vi "sub_e-top.vi"(10 "TIM_XYZ_DATA":cluster{"x":sgl, "y":sgl, "Z":sgl}[](array[cluster])=[{"x"=-0.27294323, "y"=0.40705678, "Z"=2.3861455e-08}, {"x"=-0.26954788, "y"=0.41357002, "Z"=2.3564624e-08}, {"x"=-0.26465562, "y"=0.42143202, "Z"=2.3136929e-08}, {"x"=-0.26040056, "y"=0.42853323, "Z"=2.276494e-08}, {"x"=-0.25317857, "y"=0.43833783, "Z"=2.2133573e-08}, {"x"=-0.24585162, "y"=0.4480496, "Z"=2.1493031e-08}, {"x"=-0.26621187, "y"=0.43175167, "Z"=2.327298e-08}, {"x"=-0.27206331, "y"=0.42923805, "Z"=2.378453e-08}, {"x"=-0.27573514, "y"=0.4288046, "Z"=2.4105532e-08}, {"x"=-0.278678, "y"=0.4290746, "Z"=2.4362805e-08}, {"x"=-0.27714488, "y"=0.43335915, "Z"=2.4228775e-08}, {"x"=-0.27406967, "y"=0.43893814, "Z"=2.3959931e-08}, {"x"=-0.2113174, "y"=0.496302, "Z"=1.8473955e-08}, {"x"=-0.14184111, "y"=0.558139, "Z"=1.2400144e-08}, {"x"=-0.1082447, "y"=0.58809197, "Z"=9.463053e-09}, {"x"=-0.11413979, "y"=0.5842236, "Z"=9.978417e-09}, {"x"=-0.106227584, "y"=0.59191084, "Z"=9.28671e-09}, {"x"=-0.108285144, "y"=0.5912626, "Z"=9.4665875e-09}, {"x"=-0.11113093, "y"=0.59000605, "Z"=9.715374e-09}, {"x"=-0.109310195, "y"=0.5925284, "Z"=9.556201e-09}, {"x"=-0.11373922, "y"=0.5900645, "Z"=9.943399e-09}, {"x"=-0.111896455, "y"=0.5925747, "Z"=9.7822985e-09}, {"x"=-0.110028416, "y"=0.59506035, "Z"=9.61899e-09}, {"x"=-0.11052066, "y"=0.5957018, "Z"=9.662023e-09}, {"x"=-0.11340505, "y"=0.5945407, "Z"=9.914184e-09}, {"x"=-0.11550449, "y"=0.5940075, "Z"=1.0097723e-08}, {"x"=-0.11519719, "y"=0.5952734, "Z"=1.0070858e-08}, {"x"=-0.1253962, "y"=0.5888913, "Z"=1.0962484e-08}, {"x"=-0.12348683, "y"=0.59137154, "Z"=1.0795562e-08}, {"x"=-0.001631583, "y"=0.6788433, "Z"=1.4263751e-10}, {"x"=0.0, "y"=0.68, "Z"=0.0}, {"x"=0.0, "y"=0.68, "Z"=0.0}, {"x"=0.0, "y"=0.68, "Z"=0.0}, {"x"=0.0, "y"=0.68, "Z"=0.0}, {"x"=0.0, "y"=0.68, "Z"=0.0}, {"x"=0.0, "y"=0.68, "Z"=0.0}, {"x"=-0.0016773184, "y"=0.6789107, "Z"=1.4663583e-10}, {"x"=-0.0016836267, "y"=0.67892045, "Z"=1.4718732e-10}, {"x"=-0.001689878, "y"=0.6789303, "Z"=1.4773383e-10}, {"x"=-0.0016960722, "y"=0.6789401, "Z"=1.4827534e-10}, {"x"=-0.2476714, "y"=0.5272261, "Z"=2.1652122e-08}, {"x"=-0.23916033, "y"=0.5343898, "Z"=2.090806e-08}, {"x"=-0.2365747, "y"=0.5378437, "Z"=2.0682016e-08}, {"x"=-0.23309696, "y"=0.5417726, "Z"=2.0377984e-08}, {"x"=-0.2338971, "y"=0.54313093, "Z"=2.0447935e-08}, {"x"=-0.2390194, "y"=0.54199374, "Z"=2.0895738e-08}, {"x"=-0.21635768, "y"=0.5567509, "Z"=1.8914589e-08}, {"x"=-0.23537818, "y"=0.54772335, "Z"=2.0577414e-08}, {"x"=-0.23439445, "y"=0.5500645, "Z"=2.0491413e-08}, {"x"=-0.22724964, "y"=0.5557478, "Z"=1.9866794e-08}, {"x"=-0.0017603752, "y"=0.67905074, "Z"=1.538969e-10}, {"x"=-0.0017658673, "y"=0.679061, "Z"=1.5437703e-10}, {"x"=0.0, "y"=0.68, "Z"=0.0}, {"x"=0.0, "y"=0.68, "Z"=0.0}, {"x"=0.0, "y"=0.68, "Z"=0.0}, {"x"=-0.0017872365, "y"=0.67910236, "Z"=1.5624518e-10}, {"x"=0.0, "y"=0.68, "Z"=0.0}, {"x"=0.0, "y"=0.68, "Z"=0.0}, {"x"=0.0, "y"=0.68, "Z"=0.0}, {"x"=-0.0018076382, "y"=0.6791442, "Z"=1.5802876e-10}, {"x"=-0.0018125861, "y"=0.6791547, "Z"=1.5846131e-10}, {"x"=-0.0018174726, "y"=0.67916524, "Z"=1.588885e-10}, {"x"=-0.0018222977, "y"=0.67917585, "Z"=1.5931033e-10}, {"x"=0.0, "y"=0.68, "Z"=0.0}, {"x"=0.0, "y"=0.68, "Z"=0.0}, {"x"=0.0, "y"=0.68, "Z"=0.0}, {"x"=0.0, "y"=0.68, "Z"=0.0}, {"x"=0.0, "y"=0.68, "Z"=0.0}, {"x"=0.0, "y"=0.68, "Z"=0.0}, {"x"=0.0, "y"=0.68, "Z"=0.0}, {"x"=0.0, "y"=0.68, "Z"=0.0}, {"x"=0.0, "y"=0.68, "Z"=0.0}, {"x"=0.0, "y"=0.68, "Z"=0.0}, {"x"=0.0, "y"=0.68, "Z"=0.0}, {"x"=0.0, "y"=0.68, "Z"=0.0}, {"x"=0.0, "y"=0.68, "Z"=0.0}, {"x"=0.0, "y"=0.68, "Z"=0.0}, {"x"=0.0, "y"=0.68, "Z"=0.0}, {"x"=0.0, "y"=0.68, "Z"=0.0}, {"x"=0.0, "y"=0.68, "Z"=0.0}, {"x"=0.0, "y"=0.68, "Z"=0.0}, {"x"=0.0, "y"=0.68, "Z"=0.0}, {"x"=0.0, "y"=0.68, "Z"=0.0}, {"x"=0.0, "y"=0.68, "Z"=0.0}, {"x"=0.0, "y"=0.68, "Z"=0.0}, {"x"=0.0, "y"=0.68, "Z"=0.0}, {"x"=0.0, "y"=0.68, "Z"=0.0}, {"x"=0.0, "y"=0.68, "Z"=0.0}, {"x"=0.0, "y"=0.68, "Z"=0.0}, {"x"=0.0, "y"=0.68, "Z"=0.0}, {"x"=0.0, "y"=0.68, "Z"=0.0}, {"x"=0.0, "y"=0.68, "Z"=0.0}, {"x"=0.0, "y"=0.68, "Z"=0.0}, {"x"=0.0, "y"=0.68, "Z"=0.0}, {"x"=0.0, "y"=0.68, "Z"=0.0}, {"x"=0.0, "y"=0.68, "Z"=0.0}, {"x"=0.0, "y"=0.68, "Z"=0.0}, {"x"=0.0, "y"=0.68, "Z"=0.0}, {"x"=0.0, "y"=0.68, "Z"=0.0}, {"x"=0.0, "y"=0.68, "Z"=0.0}, {"x"=0.0, "y"=0.68, "Z"=0.0}, {"x"=0.0, "y"=0.68, "Z"=0.0}, {"x"=0.0, "y"=0.68, "Z"=0.0}, {"x"=0.0, "y"=0.68, "Z"=0.0}, {"x"=0.0, "y"=0.68, "Z"=0.0}, {"x"=0.0, "y"=0.68, "Z"=0.0}, {"x"=0.0, "y"=0.68, "Z"=0.0}, {"x"=0.0, "y"=0.68, "Z"=0.0}, {"x"=0.0, "y"=0.68, "Z"=0.0}, {"x"=0.0, "y"=0.68, "Z"=0.0}, {"x"=0.0, "y"=0.68, "Z"=0.0}, {"x"=0.0, "y"=0.68, "Z"=0.0}, {"x"=0.0, "y"=0.68, "Z"=0.0}, {"x"=0.0, "y"=0.68, "Z"=0.0}, {"x"=0.0, "y"=0.68, "Z"=0.0}, {"x"=0.0, "y"=0.68, "Z"=0.0}, {"x"=0.0, "y"=0.68, "Z"=0.0}, {"x"=0.0, "y"=0.68, "Z"=0.0}, {"x"=0.0, "y"=0.68, "Z"=0.0}, {"x"=0.0, "y"=0.68, "Z"=0.0}, {"x"=0.0, "y"=0.68, "Z"=0.0}, {"x"=0.0, "y"=0.68, "Z"=0.0}, {"x"=0.0, "y"=0.68, "Z"=0.0}, {"x"=0.0, "y"=0.68, "Z"=0.0}, {"x"=0.0, "y"=0.68, "Z"=0.0}, {"x"=0.0, "y"=0.68, "Z"=0.0}, {"x"=0.0, "y"=0.68, "Z"=0.0}, {"x"=0.0, "y"=0.68, "Z"=0.0}, {"x"=0.0, "y"=0.68, "Z"=0.0}, {"x"=0.0, "y"=0.68, "Z"=0.0}, {"x"=0.0, "y"=0.68, "Z"=0.0}, {"x"=-4.297828, "y"=0.5796392, "Z"=3.7572806e-07}, {"x"=-4.2473474, "y"=0.605536, "Z"=3.713149e-07}, {"x"=-4.2397094, "y"=0.63033843, "Z"=3.7064717e-07}, {"x"=-4.235926, "y"=0.6550259, "Z"=3.7031643e-07}, {"x"=-4.232, "y"=0.67966765, "Z"=3.6997318e-07}, {"x"=-4.22593, "y"=0.70425135, "Z"=3.6944255e-07}, {"x"=-4.2197185, "y"=0.72876453, "Z"=3.688995e-07}, {"x"=-4.221363, "y"=0.75334513, "Z"=3.6904328e-07}, {"x"=-4.2148666, "y"=0.7777611, "Z"=3.6847536e-07}, {"x"=-4.203231, "y"=0.8019589, "Z"=3.674581e-07}, {"x"=-4.2054486, "y"=0.8265121, "Z"=3.67652e-07}, {"x"=-4.1975307, "y"=0.85068893, "Z"=3.669598e-07}, {"x"=-4.1914725, "y"=0.8748715, "Z"=3.6643016e-07}, {"x"=-4.1962595, "y"=0.89956415, "Z"=3.6684867e-07}, {"x"=-4.193913, "y"=0.92391264, "Z"=3.6664352e-07}, {"x"=-4.1904273, "y"=0.9481774, "Z"=3.6633878e-07}, {"x"=-4.1788206, "y"=0.97185254, "Z"=3.653241e-07}, {"x"=-4.1830354, "y"=0.9966092, "Z"=3.6569256e-07}, {"x"=-4.173149, "y"=1.020287, "Z"=3.6482828e-07}, {"x"=-4.1720953, "y"=1.0446441, "Z"=3.6473617e-07}, {"x"=-4.1699033, "y"=1.0689077, "Z"=3.6454452e-07}, {"x"=-4.164585, "y"=1.0928621, "Z"=3.640796e-07}, {"x"=-4.158135, "y"=1.1166635, "Z"=3.635157e-07}, {"x"=-4.161488, "y"=1.1415058, "Z"=3.6380885e-07}, {"x"=-4.15476, "y"=1.165242, "Z"=3.6322064e-07}, {"x"=-4.155837, "y"=1.1898898, "Z"=3.6331483e-07}, {"x"=-4.1468496, "y"=1.2132909, "Z"=3.625291e-07}, {"x"=-4.1486325, "y"=1.2380714, "Z"=3.6268497e-07}, {"x"=-4.1443257, "y"=1.2620561, "Z"=3.6230847e-07}, {"x"=-4.1388907, "y"=1.2858647, "Z"=3.6183332e-07}, {"x"=-4.1372733, "y"=1.3102322, "Z"=3.6169192e-07}, {"x"=-4.130574, "y"=1.3338196, "Z"=3.6110626e-07}, {"x"=-4.126701, "y"=1.3578367, "Z"=3.6076764e-07}, {"x"=-4.1276174, "y"=1.38267, "Z"=3.6084776e-07}, {"x"=-4.1244445, "y"=1.4068427, "Z"=3.605704e-07}, {"x"=-4.1201468, "y"=1.4308228, "Z"=3.6019466e-07}, {"x"=-4.1107955, "y"=1.4538527, "Z"=3.5937717e-07}, {"x"=-4.1150594, "y"=1.4794691, "Z"=3.5974992e-07}, {"x"=-4.1054363, "y"=1.5024114, "Z"=3.5890864e-07}, {"x"=-4.111356, "y"=1.5285027, "Z"=3.5942614e-07}, {"x"=-4.0965686, "y"=1.5503266, "Z"=3.581334e-07}, {"x"=-4.097298, "y"=1.5754232, "Z"=3.5819718e-07}, {"x"=-4.0949473, "y"=1.5999002, "Z"=3.5799167e-07}, {"x"=-4.0905013, "y"=1.6239305, "Z"=3.5760297e-07}, {"x"=-4.0917525, "y"=1.6493232, "Z"=3.5771237e-07}, {"x"=-4.087016, "y"=1.6733453, "Z"=3.572983e-07}, {"x"=-4.0869904, "y"=1.6985543, "Z"=3.5729605e-07}, {"x"=-4.0790586, "y"=1.7218165, "Z"=3.5660264e-07}, {"x"=-4.0826035, "y"=1.7480586, "Z"=3.5691252e-07}, {"x"=-4.0898447, "y"=1.7754116, "Z"=3.575456e-07}, {"x"=-4.0718303, "y"=1.7960122, "Z"=3.559707e-07}, {"x"=-4.091267, "y"=1.8269682, "Z"=3.5766993e-07}, {"x"=-4.075874, "y"=1.8482685, "Z"=3.5632422e-07}, {"x"=-4.072848, "y"=1.8730831, "Z"=3.5605967e-07}, {"x"=-4.0744605, "y"=1.8993356, "Z"=3.5620064e-07}, {"x"=-4.056779, "y"=1.9198017, "Z"=3.5465487e-07}, {"x"=-4.072409, "y"=1.9505274, "Z"=3.560213e-07}, {"x"=-4.1316504, "y"=1.9954321, "Z"=3.6120036e-07}, {"x"=-4.1895537, "y"=2.0407593, "Z"=3.662624e-07}, {"x"=-4.184415, "y"=2.0660508, "Z"=3.6581318e-07}, {"x"=-4.0578523, "y"=2.050374, "Z"=3.5474872e-07}, {"x"=-4.0356283, "y"=2.0690742, "Z"=3.5280584e-07}, {"x"=-4.032198, "y"=2.0941813, "Z"=3.5250594e-07}, {"x"=-4.0389705, "y"=2.1229963, "Z"=3.5309802e-07}, {"x"=0.0, "y"=0.68, "Z"=0.0}, {"x"=0.0, "y"=0.68, "Z"=0.0}, {"x"=0.0, "y"=0.68, "Z"=0.0}, {"x"=0.0, "y"=0.68, "Z"=0.0}, {"x"=0.0, "y"=0.68, "Z"=0.0}, {"x"=0.0, "y"=0.68, "Z"=0.0}, {"x"=0.0, "y"=0.68, "Z"=0.0}, {"x"=0.0, "y"=0.68, "Z"=0.0}, {"x"=0.0, "y"=0.68, "Z"=0.0}, {"x"=0.0, "y"=0.68, "Z"=0.0}, {"x"=0.0, "y"=0.68, "Z"=0.0}, {"x"=0.0, "y"=0.68, "Z"=0.0}, {"x"=0.0, "y"=0.68, "Z"=0.0}, {"x"=0.0, "y"=0.68, "Z"=0.0}, {"x"=0.0, "y"=0.68, "Z"=0.0}, {"x"=0.0, "y"=0.68, "Z"=0.0}, {"x"=0.0, "y"=0.68, "Z"=0.0}, {"x"=0.0, "y"=0.68, "Z"=0.0}, {"x"=0.0, "y"=0.68, "Z"=0.0}, {"x"=0.0, "y"=0.68, "Z"=0.0}, {"x"=0.0, "y"=0.68, "Z"=0.0}, {"x"=0.0, "y"=0.68, "Z"=0.0}, {"x"=0.0, "y"=0.68, "Z"=0.0}, {"x"=0.0, "y"=0.68, "Z"=0.0}, {"x"=0.0, "y"=0.68, "Z"=0.0}, {"x"=-0.0017605242, "y"=0.680949, "Z"=1.5390991e-10}, {"x"=-1.5162977, "y"=1.5087492, "Z"=1.3255895e-07}, {"x"=-1.5044535, "y"=1.5136783, "Z"=1.315235e-07}, {"x"=-1.4891163, "y"=1.5165384, "Z"=1.3018268e-07}, {"x"=-1.474666, "y"=1.5197434, "Z"=1.289194e-07}, {"x"=-1.4758188, "y"=1.5318068, "Z"=1.2902018e-07}, {"x"=-1.48206, "y"=1.5469414, "Z"=1.2956579e-07}, {"x"=-1.5802177, "y"=1.6167395, "Z"=1.3814702e-07}, {"x"=-1.7170429, "y"=1.7113936, "Z"=1.5010866e-07}, {"x"=-1.7204106, "y"=1.7270832, "Z"=1.5040307e-07}, {"x"=-1.7219511, "y"=1.7417972, "Z"=1.5053774e-07}, {"x"=-1.7191378, "y"=1.7539153, "Z"=1.502918e-07}, {"x"=0.0, "y"=0.68, "Z"=0.0}, {"x"=0.0, "y"=0.68, "Z"=0.0}, {"x"=0.0, "y"=0.68, "Z"=0.0}, {"x"=0.0, "y"=0.68, "Z"=0.0}, {"x"=0.0, "y"=0.68, "Z"=0.0}, {"x"=0.0, "y"=0.68, "Z"=0.0}, {"x"=0.0, "y"=0.68, "Z"=0.0}, {"x"=0.0, "y"=0.68, "Z"=0.0}, {"x"=0.0, "y"=0.68, "Z"=0.0}, {"x"=0.0, "y"=0.68, "Z"=0.0}, {"x"=0.0, "y"=0.68, "Z"=0.0}, {"x"=0.0, "y"=0.68, "Z"=0.0}, {"x"=0.0, "y"=0.68, "Z"=0.0}, {"x"=0.0, "y"=0.68, "Z"=0.0}, {"x"=0.0, "y"=0.68, "Z"=0.0}, {"x"=0.0, "y"=0.68, "Z"=0.0}, {"x"=0.0, "y"=0.68, "Z"=0.0}, {"x"=0.0, "y"=0.68, "Z"=0.0}, {"x"=0.0, "y"=0.68, "Z"=0.0}, {"x"=0.0, "y"=0.68, "Z"=0.0}, {"x"=0.0, "y"=0.68, "Z"=0.0}, {"x"=0.0, "y"=0.68, "Z"=0.0}, {"x"=0.0, "y"=0.68, "Z"=0.0}, {"x"=0.0, "y"=0.68, "Z"=0.0}, {"x"=0.0, "y"=0.68, "Z"=0.0}, {"x"=0.0, "y"=0.68, "Z"=0.0}, {"x"=0.0, "y"=0.68, "Z"=0.0}, {"x"=0.0, "y"=0.68, "Z"=0.0}, {"x"=0.0, "y"=0.68, "Z"=0.0}, {"x"=0.0, "y"=0.68, "Z"=0.0}, {"x"=0.0, "y"=0.68, "Z"=0.0}, {"x"=0.0, "y"=0.68, "Z"=0.0}, {"x"=-0.0014629168, "y"=0.68136376, "Z"=1.2789225e-10}, {"x"=-4.667508, "y"=5.0822067, "Z"=4.0804653e-07}, {"x"=-4.7156153, "y"=5.1796994, "Z"=4.1225218e-07}, {"x"=-4.6836047, "y"=5.2014985, "Z"=4.0945372e-07}, {"x"=-4.668669, "y"=5.2398467, "Z"=4.0814803e-07}, {"x"=-4.633529, "y"=5.2584934, "Z"=4.0507598e-07}, {"x"=-4.5403385, "y"=5.218912, "Z"=3.96929e-07}, {"x"=-4.4948745, "y"=5.2260475, "Z"=3.929544e-07}, {"x"=-4.451579, "y"=5.234954, "Z"=3.891694e-07}, {"x"=-4.399995, "y"=5.23488, "Z"=3.8465976e-07}, {"x"=-4.375496, "y"=5.262568, "Z"=3.82518e-07}, {"x"=-4.3570004, "y"=5.296671, "Z"=3.8090107e-07}, {"x"=-4.3819118, "y"=5.3775125, "Z"=3.8307888e-07}, {"x"=-4.416874, "y"=5.4705615, "Z"=3.8613538e-07}, {"x"=-4.337067, "y"=5.439261, "Z"=3.7915845e-07}, {"x"=-4.2229753, "y"=5.3685584, "Z"=3.6918422e-07}, {"x"=0.0, "y"=0.68, "Z"=0.0}, {"x"=0.0, "y"=0.68, "Z"=0.0}, {"x"=0.0, "y"=0.68, "Z"=0.0}, {"x"=0.0, "y"=0.68, "Z"=0.0}, {"x"=0.0, "y"=0.68, "Z"=0.0}, {"x"=0.0, "y"=0.68, "Z"=0.0}, {"x"=0.0, "y"=0.68, "Z"=0.0}, {"x"=0.0, "y"=0.68, "Z"=0.0}, {"x"=0.0, "y"=0.68, "Z"=0.0}, {"x"=0.0, "y"=0.68, "Z"=0.0}, {"x"=0.0, "y"=0.68, "Z"=0.0}, {"x"=0.0, "y"=0.68, "Z"=0.0}, {"x"=0.0, "y"=0.68, "Z"=0.0}, {"x"=0.0, "y"=0.68, "Z"=0.0}, {"x"=0.0, "y"=0.68, "Z"=0.0}, {"x"=0.0, "y"=0.68, "Z"=0.0}, {"x"=0.0, "y"=0.68, "Z"=0.0}, {"x"=0.0, "y"=0.68, "Z"=0.0}, {"x"=0.0, "y"=0.68, "Z"=0.0}, {"x"=0.0, "y"=0.68, "Z"=0.0}, {"x"=0.0, "y"=0.68, "Z"=0.0}, {"x"=0.0, "y"=0.68, "Z"=0.0}, {"x"=0.0, "y"=0.68, "Z"=0.0}, {"x"=0.0, "y"=0.68, "Z"=0.0}, {"x"=0.0, "y"=0.68, "Z"=0.0}, {"x"=0.0, "y"=0.68, "Z"=0.0}, {"x"=0.0, "y"=0.68, "Z"=0.0}, {"x"=0.0, "y"=0.68, "Z"=0.0}, {"x"=0.0, "y"=0.68, "Z"=0.0}, {"x"=-1.6903987, "y"=3.3841217, "Z"=1.4777935e-07}, {"x"=-1.6174006, "y"=3.3011477, "Z"=1.4139765e-07}, {"x"=-1.5958836, "y"=3.3002634, "Z"=1.3951657e-07}, {"x"=-1.5764925, "y"=3.302646, "Z"=1.3782136e-07}, {"x"=-1.5566177, "y"=3.3040316, "Z"=1.3608384e-07}, {"x"=-1.546379, "y"=3.3216724, "Z"=1.3518874e-07}, {"x"=-1.5319861, "y"=3.3323553, "Z"=1.3393048e-07}, {"x"=-1.520987, "y"=3.3490415, "Z"=1.329689e-07}, {"x"=0.0, "y"=0.68, "Z"=0.0}, {"x"=0.0, "y"=0.68, "Z"=0.0}, {"x"=-4.2809734, "y"=8.506718, "Z"=3.742546e-07}, {"x"=-4.2310987, "y"=8.523567, "Z"=3.698944e-07}, {"x"=-4.1666145, "y"=8.512733, "Z"=3.64257e-07}, {"x"=0.0, "y"=0.68, "Z"=0.0}, {"x"=0.0, "y"=0.68, "Z"=0.0}, {"x"=0.0, "y"=0.68, "Z"=0.0}, {"x"=0.0, "y"=0.68, "Z"=0.0}, {"x"=0.0, "y"=0.68, "Z"=0.0}, {"x"=0.0, "y"=0.68, "Z"=0.0}, {"x"=0.0, "y"=0.68, "Z"=0.0}, {"x"=0.0, "y"=0.68, "Z"=0.0}, {"x"=0.0, "y"=0.68, "Z"=0.0}, {"x"=0.0, "y"=0.68, "Z"=0.0}, {"x"=0.0, "y"=0.68, "Z"=0.0}, {"x"=0.0, "y"=0.68, "Z"=0.0}, {"x"=0.0, "y"=0.68, "Z"=0.0}, {"x"=0.0, "y"=0.68, "Z"=0.0}, {"x"=0.0, "y"=0.68, "Z"=0.0}, {"x"=0.0, "y"=0.68, "Z"=0.0}, {"x"=0.0, "y"=0.68, "Z"=0.0}, {"x"=0.0, "y"=0.68, "Z"=0.0}, {"x"=0.0, "y"=0.68, "Z"=0.0}, {"x"=0.0, "y"=0.68, "Z"=0.0}, {"x"=0.0, "y"=0.68, "Z"=0.0}, {"x"=0.0, "y"=0.68, "Z"=0.0}, {"x"=0.0, "y"=0.68, "Z"=0.0}, {"x"=0.0, "y"=0.68, "Z"=0.0}, {"x"=0.0, "y"=0.68, "Z"=0.0}, {"x"=0.0, "y"=0.68, "Z"=0.0}, {"x"=0.0, "y"=0.68, "Z"=0.0}, {"x"=0.0, "y"=0.68, "Z"=0.0}, {"x"=-3.8586884, "y"=12.31693, "Z"=3.3733724e-07}, {"x"=-3.769903, "y"=12.274511, "Z"=3.2957539e-07}, {"x"=-3.7087693, "y"=12.316254, "Z"=3.242309e-07}, {"x"=-3.65801, "y"=12.392039, "Z"=3.197934e-07}, {"x"=-3.6000571, "y"=12.446589, "Z"=3.14727e-07}, {"x"=-3.5338442, "y"=12.474996, "Z"=3.0893847e-07}, {"x"=-0.0005628476, "y"=0.68191916, "Z"=4.92057e-11}, {"x"=0.0, "y"=0.68, "Z"=0.0}, {"x"=0.0, "y"=0.68, "Z"=0.0}, {"x"=0.0, "y"=0.68, "Z"=0.0}, {"x"=0.0, "y"=0.68, "Z"=0.0}, {"x"=0.0, "y"=0.68, "Z"=0.0}, {"x"=0.0, "y"=0.68, "Z"=0.0}, {"x"=0.0, "y"=0.68, "Z"=0.0}, {"x"=0.0, "y"=0.68, "Z"=0.0}, {"x"=0.0, "y"=0.68, "Z"=0.0}, {"x"=0.0, "y"=0.68, "Z"=0.0}, {"x"=0.0, "y"=0.68, "Z"=0.0}, {"x"=0.0, "y"=0.68, "Z"=0.0}, {"x"=0.0, "y"=0.68, "Z"=0.0}, {"x"=0.0, "y"=0.68, "Z"=0.0}, {"x"=0.0, "y"=0.68, "Z"=0.0}, {"x"=0.0, "y"=0.68, "Z"=0.0}, {"x"=0.0, "y"=0.68, "Z"=0.0}, {"x"=0.0, "y"=0.68, "Z"=0.0}, {"x"=0.0, "y"=0.68, "Z"=0.0}, {"x"=0.0, "y"=0.68, "Z"=0.0}, {"x"=0.0, "y"=0.68, "Z"=0.0}, {"x"=0.0, "y"=0.68, "Z"=0.0}, {"x"=0.0, "y"=0.68, "Z"=0.0}, {"x"=0.0, "y"=0.68, "Z"=0.0}, {"x"=0.0, "y"=0.68, "Z"=0.0}, {"x"=0.0, "y"=0.68, "Z"=0.0}, {"x"=0.0, "y"=0.68, "Z"=0.0}, {"x"=0.0, "y"=0.68, "Z"=0.0}, {"x"=0.0, "y"=0.68, "Z"=0.0}, {"x"=0.0, "y"=0.68, "Z"=0.0}, {"x"=0.0, "y"=0.68, "Z"=0.0}, {"x"=0.0, "y"=0.68, "Z"=0.0}, {"x"=0.0, "y"=0.68, "Z"=0.0}, {"x"=0.0, "y"=0.68, "Z"=0.0}, {"x"=0.0, "y"=0.68, "Z"=0.0}, {"x"=0.0, "y"=0.68, "Z"=0.0}, {"x"=0.0, "y"=0.68, "Z"=0.0}, {"x"=0.0, "y"=0.68, "Z"=0.0}, {"x"=0.0, "y"=0.68, "Z"=0.0}, {"x"=0.0, "y"=0.68, "Z"=0.0}, {"x"=0.0, "y"=0.68, "Z"=0.0}, {"x"=0.0, "y"=0.68, "Z"=0.0}, {"x"=0.0, "y"=0.68, "Z"=0.0}, {"x"=0.0, "y"=0.68, "Z"=0.0}, {"x"=0.0, "y"=0.68, "Z"=0.0}, {"x"=0.0, "y"=0.68, "Z"=0.0}, {"x"=0.0, "y"=0.68, "Z"=0.0}, {"x"=0.0, "y"=0.68, "Z"=0.0}, {"x"=0.0, "y"=0.68, "Z"=0.0}, {"x"=0.0, "y"=0.68, "Z"=0.0}, {"x"=0.0, "y"=0.68, "Z"=0.0}, {"x"=0.0, "y"=0.68, "Z"=0.0}, {"x"=0.0, "y"=0.68, "Z"=0.0}, {"x"=0.0, "y"=0.68, "Z"=0.0}, {"x"=0.0, "y"=0.68, "Z"=0.0}, {"x"=0.0, "y"=0.68, "Z"=0.0}, {"x"=0.0, "y"=0.68, "Z"=0.0}, {"x"=0.0, "y"=0.68, "Z"=0.0}, {"x"=0.0, "y"=0.68, "Z"=0.0}, {"x"=0.0, "y"=0.68, "Z"=0.0}, {"x"=0.0, "y"=0.68, "Z"=0.0}, {"x"=0.0, "y"=0.68, "Z"=0.0}, {"x"=0.0, "y"=0.68, "Z"=0.0}, {"x"=0.0, "y"=0.68, "Z"=0.0}, {"x"=0.0, "y"=0.68, "Z"=0.0}, {"x"=0.0, "y"=0.68, "Z"=0.0}, {"x"=0.0, "y"=0.68, "Z"=0.0}, {"x"=0.0, "y"=0.68, "Z"=0.0}, {"x"=0.0, "y"=0.68, "Z"=0.0}, {"x"=0.0, "y"=0.68, "Z"=0.0}, {"x"=0.0, "y"=0.68, "Z"=0.0}, {"x"=0.0, "y"=0.68, "Z"=0.0}, {"x"=0.0, "y"=0.68, "Z"=0.0}, {"x"=0.0, "y"=0.68, "Z"=0.0}, {"x"=0.0, "y"=0.68, "Z"=0.0}, {"x"=0.0, "y"=0.68, "Z"=0.0}, {"x"=0.0, "y"=0.68, "Z"=0.0}, {"x"=0.0, "y"=0.68, "Z"=0.0}, {"x"=0.0, "y"=0.68, "Z"=0.0}, {"x"=0.0, "y"=0.68, "Z"=0.0}, {"x"=0.0, "y"=0.68, "Z"=0.0}, {"x"=0.0, "y"=0.68, "Z"=0.0}, {"x"=0.0, "y"=0.68, "Z"=0.0}, {"x"=0.0, "y"=0.68, "Z"=0.0}, {"x"=0.0, "y"=0.68, "Z"=0.0}, {"x"=0.0, "y"=0.68, "Z"=0.0}, {"x"=0.0, "y"=0.68, "Z"=0.0}, {"x"=0.0, "y"=0.68, "Z"=0.0}, {"x"=0.0, "y"=0.68, "Z"=0.0}, {"x"=0.0, "y"=0.68, "Z"=0.0}, {"x"=0.0, "y"=0.68, "Z"=0.0}, {"x"=0.0, "y"=0.68, "Z"=0.0}, {"x"=0.0, "y"=0.68, "Z"=0.0}, {"x"=0.0, "y"=0.68, "Z"=0.0}, {"x"=0.6654722, "y"=3.1095078, "Z"=-5.8177427e-08}, {"x"=0.6709606, "y"=3.0747821, "Z"=-5.865724e-08}, {"x"=0.67799544, "y"=3.0468051, "Z"=-5.9272246e-08}, {"x"=0.69119006, "y"=3.0409017, "Z"=-6.0425755e-08}, {"x"=0.70519865, "y"=3.0377991, "Z"=-6.1650425e-08}, {"x"=0.72007084, "y"=3.0374825, "Z"=-6.295059e-08}, {"x"=0.7346655, "y"=3.0361178, "Z"=-6.42265e-08}, {"x"=0.753817, "y"=3.0489569, "Z"=-6.590078e-08}, {"x"=0.77098125, "y"=3.054994, "Z"=-6.7401324e-08}, {"x"=0.0, "y"=0.68, "Z"=0.0}, {"x"=0.0, "y"=0.68, "Z"=0.0}, {"x"=0.0, "y"=0.68, "Z"=0.0}, {"x"=0.0, "y"=0.68, "Z"=0.0}, {"x"=0.0, "y"=0.68, "Z"=0.0}, {"x"=0.0, "y"=0.68, "Z"=0.0}, {"x"=0.0, "y"=0.68, "Z"=0.0}, {"x"=0.0, "y"=0.68, "Z"=0.0}, {"x"=0.0, "y"=0.68, "Z"=0.0}, {"x"=0.0, "y"=0.68, "Z"=0.0}, {"x"=0.0, "y"=0.68, "Z"=0.0}, {"x"=0.8939538, "y"=2.89436, "Z"=-7.815192e-08}, {"x"=0.903782, "y"=2.8817217, "Z"=-7.901113e-08}, {"x"=0.9092573, "y"=2.8588924, "Z"=-7.9489794e-08}, {"x"=0.9133263, "y"=2.8333127, "Z"=-7.984552e-08}, {"x"=0.9234621, "y"=2.8224535, "Z"=-8.073162e-08}, {"x"=0.93550825, "y"=2.8161294, "Z"=-8.178473e-08}, {"x"=0.9458862, "y"=2.806083, "Z"=-8.2692e-08}, {"x"=0.96688557, "y"=2.8196814, "Z"=-8.452782e-08}, {"x"=0.98682356, "y"=2.8303802, "Z"=-8.627086e-08}, {"x"=1.0001607, "y"=2.8264163, "Z"=-8.7436824e-08}, {"x"=0.0, "y"=0.68, "Z"=0.0}, {"x"=0.0, "y"=0.68, "Z"=0.0}, {"x"=0.0, "y"=0.68, "Z"=0.0}, {"x"=0.0, "y"=0.68, "Z"=0.0}, {"x"=0.0, "y"=0.68, "Z"=0.0}, {"x"=0.0, "y"=0.68, "Z"=0.0}, {"x"=0.0, "y"=0.68, "Z"=0.0}, {"x"=0.0, "y"=0.68, "Z"=0.0}, {"x"=0.0, "y"=0.68, "Z"=0.0}, {"x"=0.0, "y"=0.68, "Z"=0.0}, {"x"=0.0, "y"=0.68, "Z"=0.0}, {"x"=0.0, "y"=0.68, "Z"=0.0}, {"x"=0.0, "y"=0.68, "Z"=0.0}, {"x"=0.0, "y"=0.68, "Z"=0.0}, {"x"=0.0, "y"=0.68, "Z"=0.0}, {"x"=0.0, "y"=0.68, "Z"=0.0}, {"x"=0.0, "y"=0.68, "Z"=0.0}, {"x"=0.0, "y"=0.68, "Z"=0.0}, {"x"=0.0, "y"=0.68, "Z"=0.0}, {"x"=0.0, "y"=0.68, "Z"=0.0}, {"x"=0.0, "y"=0.68, "Z"=0.0}, {"x"=0.0, "y"=0.68, "Z"=0.0}, {"x"=0.0, "y"=0.68, "Z"=0.0}, {"x"=0.0, "y"=0.68, "Z"=0.0}, {"x"=0.0, "y"=0.68, "Z"=0.0}, {"x"=0.0, "y"=0.68, "Z"=0.0}, {"x"=0.0, "y"=0.68, "Z"=0.0}, {"x"=0.0, "y"=0.68, "Z"=0.0}, {"x"=0.0, "y"=0.68, "Z"=0.0}, {"x"=0.0, "y"=0.68, "Z"=0.0}, {"x"=0.0, "y"=0.68, "Z"=0.0}, {"x"=0.0, "y"=0.68, "Z"=0.0}, {"x"=0.0, "y"=0.68, "Z"=0.0}, {"x"=0.0, "y"=0.68, "Z"=0.0}, {"x"=0.0, "y"=0.68, "Z"=0.0}, {"x"=0.0, "y"=0.68, "Z"=0.0}, {"x"=0.0, "y"=0.68, "Z"=0.0}, {"x"=0.0, "y"=0.68, "Z"=0.0}, {"x"=0.0, "y"=0.68, "Z"=0.0}, {"x"=0.0, "y"=0.68, "Z"=0.0}, {"x"=0.0, "y"=0.68, "Z"=0.0}, {"x"=0.0, "y"=0.68, "Z"=0.0}, {"x"=0.0, "y"=0.68, "Z"=0.0}, {"x"=0.0, "y"=0.68, "Z"=0.0}, {"x"=0.0, "y"=0.68, "Z"=0.0}, {"x"=0.0, "y"=0.68, "Z"=0.0}, {"x"=0.0, "y"=0.68, "Z"=0.0}, {"x"=0.0, "y"=0.68, "Z"=0.0}, {"x"=0.0, "y"=0.68, "Z"=0.0}, {"x"=0.0, "y"=0.68, "Z"=0.0}, {"x"=0.0, "y"=0.68, "Z"=0.0}, {"x"=0.0, "y"=0.68, "Z"=0.0}, {"x"=0.0, "y"=0.68, "Z"=0.0}, {"x"=0.0, "y"=0.68, "Z"=0.0}, {"x"=0.0, "y"=0.68, "Z"=0.0}, {"x"=0.0, "y"=0.68, "Z"=0.0}, {"x"=0.0, "y"=0.68, "Z"=0.0}, {"x"=0.0, "y"=0.68, "Z"=0.0}, {"x"=0.0, "y"=0.68, "Z"=0.0}, {"x"=0.0, "y"=0.68, "Z"=0.0}, {"x"=0.0, "y"=0.68, "Z"=0.0}, {"x"=0.0, "y"=0.68, "Z"=0.0}, {"x"=0.0, "y"=0.68, "Z"=0.0}, {"x"=0.0, "y"=0.68, "Z"=0.0}, {"x"=0.0, "y"=0.68, "Z"=0.0}, {"x"=0.0, "y"=0.68, "Z"=0.0}, {"x"=0.0, "y"=0.68, "Z"=0.0}, {"x"=7.5883055, "y"=7.597329, "Z"=-6.633907e-07}, {"x"=7.648475, "y"=7.5711427, "Z"=-6.6865096e-07}, {"x"=7.771329, "y"=7.600353, "Z"=-6.793912e-07}, {"x"=0.0, "y"=0.68, "Z"=0.0}, {"x"=0.0, "y"=0.68, "Z"=0.0}, {"x"=0.0, "y"=0.68, "Z"=0.0}, {"x"=0.0, "y"=0.68, "Z"=0.0}, {"x"=0.0, "y"=0.68, "Z"=0.0}, {"x"=0.0, "y"=0.68, "Z"=0.0}, {"x"=0.0, "y"=0.68, "Z"=0.0}, {"x"=0.0, "y"=0.68, "Z"=0.0}, {"x"=0.0, "y"=0.68, "Z"=0.0}, {"x"=0.0, "y"=0.68, "Z"=0.0}, {"x"=0.0, "y"=0.68, "Z"=0.0}, {"x"=0.0, "y"=0.68, "Z"=0.0}, {"x"=0.0, "y"=0.68, "Z"=0.0}, {"x"=0.0, "y"=0.68, "Z"=0.0}, {"x"=0.0, "y"=0.68, "Z"=0.0}, {"x"=0.0, "y"=0.68, "Z"=0.0}, {"x"=0.0, "y"=0.68, "Z"=0.0}, {"x"=0.0, "y"=0.68, "Z"=0.0}, {"x"=0.0, "y"=0.68, "Z"=0.0}, {"x"=0.0, "y"=0.68, "Z"=0.0}, {"x"=0.0, "y"=0.68, "Z"=0.0}, {"x"=0.0, "y"=0.68, "Z"=0.0}, {"x"=0.0, "y"=0.68, "Z"=0.0}, {"x"=0.0, "y"=0.68, "Z"=0.0}, {"x"=0.0, "y"=0.68, "Z"=0.0}, {"x"=0.0, "y"=0.68, "Z"=0.0}, {"x"=0.0, "y"=0.68, "Z"=0.0}, {"x"=0.0, "y"=0.68, "Z"=0.0}, {"x"=0.0, "y"=0.68, "Z"=0.0}, {"x"=0.0, "y"=0.68, "Z"=0.0}, {"x"=0.0, "y"=0.68, "Z"=0.0}, {"x"=0.0, "y"=0.68, "Z"=0.0}, {"x"=0.0, "y"=0.68, "Z"=0.0}, {"x"=0.0, "y"=0.68, "Z"=0.0}, {"x"=0.0, "y"=0.68, "Z"=0.0}, {"x"=0.0, "y"=0.68, "Z"=0.0}, {"x"=0.0, "y"=0.68, "Z"=0.0}, {"x"=0.0, "y"=0.68, "Z"=0.0}, {"x"=0.0, "y"=0.68, "Z"=0.0}, {"x"=0.0, "y"=0.68, "Z"=0.0}, {"x"=0.0, "y"=0.68, "Z"=0.0}, {"x"=0.0, "y"=0.68, "Z"=0.0}, {"x"=0.0, "y"=0.68, "Z"=0.0}, {"x"=0.0, "y"=0.68, "Z"=0.0}, {"x"=0.0, "y"=0.68, "Z"=0.0}, {"x"=0.0, "y"=0.68, "Z"=0.0}, {"x"=0.0017972834, "y"=0.6808774, "Z"=-1.5712351e-10}, {"x"=0.0, "y"=0.68, "Z"=0.0}, {"x"=0.0, "y"=0.68, "Z"=0.0}, {"x"=7.49032, "y"=4.175977, "Z"=-6.548246e-07}, {"x"=7.4360247, "y"=4.0980983, "Z"=-6.5007794e-07}, {"x"=7.433918, "y"=4.044887, "Z"=-6.4989376e-07}, {"x"=7.3821206, "y"=3.9698355, "Z"=-6.453655e-07}, {"x"=7.372745, "y"=3.9143832, "Z"=-6.445458e-07}, {"x"=7.2849383, "y"=3.8254573, "Z"=-6.368695e-07}, {"x"=7.304033, "y"=3.7834175, "Z"=-6.3853884e-07}, {"x"=7.3256526, "y"=3.7424192, "Z"=-6.404289e-07}, {"x"=7.3322453, "y"=3.695189, "Z"=-6.410053e-07}, {"x"=7.2801323, "y"=3.624365, "Z"=-6.364494e-07}, {"x"=7.2451005, "y"=3.5612717, "Z"=-6.333868e-07}, {"x"=7.201201, "y"=3.495409, "Z"=-6.29549e-07}, {"x"=7.1633167, "y"=3.4326663, "Z"=-6.26237e-07}, {"x"=7.1361737, "y"=3.3746996, "Z"=-6.2386414e-07}, {"x"=7.1282897, "y"=3.3244464, "Z"=-6.2317486e-07}, {"x"=7.0806007, "y"=3.2599974, "Z"=-6.190058e-07}, {"x"=7.073834, "y"=3.2110164, "Z"=-6.184142e-07}, {"x"=7.0959854, "y"=3.1724753, "Z"=-6.2035076e-07}, {"x"=7.0678215, "y"=3.116489, "Z"=-6.178886e-07}, {"x"=7.089453, "y"=3.0778964, "Z"=-6.197797e-07}, {"x"=7.0966387, "y"=3.0344112, "Z"=-6.2040783e-07}, {"x"=7.07598, "y"=2.9819522, "Z"=-6.1860186e-07}, {"x"=7.080677, "y"=2.9380167, "Z"=-6.1901244e-07}, {"x"=7.0602856, "y"=2.8863494, "Z"=-6.172298e-07}, {"x"=7.0806503, "y"=2.847583, "Z"=-6.190101e-07}, {"x"=7.10655, "y"=2.8103774, "Z"=-6.2127435e-07}, {"x"=7.1456895, "y"=2.7768855, "Z"=-6.2469604e-07}, {"x"=7.1212425, "y"=2.724795, "Z"=-6.225588e-07}, {"x"=7.1349425, "y"=2.6838758, "Z"=-6.237565e-07}, {"x"=7.1377997, "y"=2.6399539, "Z"=-6.2400625e-07}, {"x"=7.196406, "y"=2.6110985, "Z"=-6.291298e-07}, {"x"=7.2558837, "y"=2.5818808, "Z"=-6.343295e-07}, {"x"=7.268762, "y"=2.5401359, "Z"=-6.3545536e-07}, {"x"=7.2814, "y"=2.4983053, "Z"=-6.3656023e-07}, {"x"=7.3122582, "y"=2.460887, "Z"=-6.392579e-07}, {"x"=7.345845, "y"=2.4238636, "Z"=-6.421942e-07}, {"x"=7.4084764, "y"=2.393269, "Z"=-6.476696e-07}, {"x"=7.454414, "y"=2.3582706, "Z"=-6.516856e-07}, {"x"=7.47968, "y"=2.3183022, "Z"=-6.538944e-07}, {"x"=7.5145135, "y"=2.2801793, "Z"=-6.569396e-07}, {"x"=7.5227156, "y"=2.2362366, "Z"=-6.576567e-07}, {"x"=7.5708585, "y"=2.2003248, "Z"=-6.6186544e-07}, {"x"=7.7366233, "y"=2.1868463, "Z"=-6.763571e-07}, {"x"=7.7658935, "y"=2.1457105, "Z"=-6.7891597e-07}, {"x"=7.888399, "y"=2.1213603, "Z"=-6.896258e-07}, {"x"=8.009895, "y"=2.0954602, "Z"=-7.002473e-07}, {"x"=8.012079, "y"=2.0478315, "Z"=-7.004382e-07}, {"x"=8.0090475, "y"=1.999413, "Z"=-7.001732e-07}, {"x"=0.0019752586, "y"=0.68031365, "Z"=-1.7268259e-10}, {"x"=0.0, "y"=0.68, "Z"=0.0}, {"x"=0.0, "y"=0.68, "Z"=0.0}, {"x"=0.0, "y"=0.68, "Z"=0.0}, {"x"=0.0, "y"=0.68, "Z"=0.0}, {"x"=0.0, "y"=0.68, "Z"=0.0}, {"x"=0.0, "y"=0.68, "Z"=0.0}, {"x"=0.0, "y"=0.68, "Z"=0.0}, {"x"=0.0, "y"=0.68, "Z"=0.0}, {"x"=0.0, "y"=0.68, "Z"=0.0}, {"x"=0.0, "y"=0.68, "Z"=0.0}, {"x"=0.0, "y"=0.68, "Z"=0.0}, {"x"=0.0, "y"=0.68, "Z"=0.0}, {"x"=0.0, "y"=0.68, "Z"=0.0}, {"x"=0.0, "y"=0.68, "Z"=0.0}, {"x"=0.0, "y"=0.68, "Z"=0.0}, {"x"=0.0, "y"=0.68, "Z"=0.0}, {"x"=0.0, "y"=0.68, "Z"=0.0}, {"x"=0.0, "y"=0.68, "Z"=0.0}, {"x"=0.0, "y"=0.68, "Z"=0.0}, {"x"=0.0, "y"=0.68, "Z"=0.0}, {"x"=0.0, "y"=0.68, "Z"=0.0}, {"x"=0.0, "y"=0.68, "Z"=0.0}, {"x"=0.0, "y"=0.68, "Z"=0.0}, {"x"=0.0, "y"=0.68, "Z"=0.0}, {"x"=0.0, "y"=0.68, "Z"=0.0}, {"x"=0.0, "y"=0.68, "Z"=0.0}, {"x"=0.0, "y"=0.68, "Z"=0.0}, {"x"=0.0, "y"=0.68, "Z"=0.0}, {"x"=0.0, "y"=0.68, "Z"=0.0}, {"x"=0.0, "y"=0.68, "Z"=0.0}, {"x"=0.0, "y"=0.68, "Z"=0.0}, {"x"=0.0, "y"=0.68, "Z"=0.0}, {"x"=0.0, "y"=0.68, "Z"=0.0}, {"x"=0.0, "y"=0.68, "Z"=0.0}, {"x"=0.0, "y"=0.68, "Z"=0.0}, {"x"=0.0, "y"=0.68, "Z"=0.0}, {"x"=0.0, "y"=0.68, "Z"=0.0}, {"x"=0.0, "y"=0.68, "Z"=0.0}, {"x"=0.0, "y"=0.68, "Z"=0.0}, {"x"=0.0, "y"=0.68, "Z"=0.0}, {"x"=0.0, "y"=0.68, "Z"=0.0}, {"x"=0.0, "y"=0.68, "Z"=0.0}, {"x"=0.0, "y"=0.68, "Z"=0.0}, {"x"=0.0, "y"=0.68, "Z"=0.0}, {"x"=0.0, "y"=0.68, "Z"=0.0}, {"x"=0.0, "y"=0.68, "Z"=0.0}, {"x"=0.0, "y"=0.68, "Z"=0.0}, {"x"=0.0, "y"=0.68, "Z"=0.0}, {"x"=0.0, "y"=0.68, "Z"=0.0}, {"x"=0.0, "y"=0.68, "Z"=0.0}, {"x"=0.0, "y"=0.68, "Z"=0.0}, {"x"=0.0, "y"=0.68, "Z"=0.0}, {"x"=0.0, "y"=0.68, "Z"=0.0}, {"x"=0.0, "y"=0.68, "Z"=0.0}, {"x"=0.0, "y"=0.68, "Z"=0.0}, {"x"=0.0, "y"=0.68, "Z"=0.0}, {"x"=0.0, "y"=0.68, "Z"=0.0}, {"x"=0.0, "y"=0.68, "Z"=0.0}, {"x"=0.0, "y"=0.68, "Z"=0.0}, {"x"=0.0, "y"=0.68, "Z"=0.0}, {"x"=0.0, "y"=0.68, "Z"=0.0}, {"x"=0.0, "y"=0.68, "Z"=0.0}, {"x"=0.0, "y"=0.68, "Z"=0.0}, {"x"=0.0, "y"=0.68, "Z"=0.0}, {"x"=0.0, "y"=0.68, "Z"=0.0}, {"x"=0.0, "y"=0.68, "Z"=0.0}, {"x"=0.0, "y"=0.68, "Z"=0.0}, {"x"=0.0, "y"=0.68, "Z"=0.0}, {"x"=0.0, "y"=0.68, "Z"=0.0}, {"x"=0.0, "y"=0.68, "Z"=0.0}, {"x"=0.0, "y"=0.68, "Z"=0.0}, {"x"=0.0, "y"=0.68, "Z"=0.0}, {"x"=0.0, "y"=0.68, "Z"=0.0}, {"x"=0.0, "y"=0.68, "Z"=0.0}, {"x"=0.0, "y"=0.68, "Z"=0.0}, {"x"=0.0, "y"=0.68, "Z"=0.0}, {"x"=0.0, "y"=0.68, "Z"=0.0}, {"x"=0.0, "y"=0.68, "Z"=0.0}, {"x"=0.0, "y"=0.68, "Z"=0.0}, {"x"=0.0, "y"=0.68, "Z"=0.0}, {"x"=0.0, "y"=0.68, "Z"=0.0}, {"x"=0.0, "y"=0.68, "Z"=0.0}, {"x"=0.0, "y"=0.68, "Z"=0.0}, {"x"=0.0, "y"=0.68, "Z"=0.0}, {"x"=0.0, "y"=0.68, "Z"=0.0}, {"x"=0.0, "y"=0.68, "Z"=0.0}, {"x"=0.0, "y"=0.68, "Z"=0.0}, {"x"=0.0, "y"=0.68, "Z"=0.0}, {"x"=0.0, "y"=0.68, "Z"=0.0}, {"x"=0.0, "y"=0.68, "Z"=0.0}, {"x"=0.0, "y"=0.68, "Z"=0.0}, {"x"=0.0, "y"=0.68, "Z"=0.0}, {"x"=0.0, "y"=0.68, "Z"=0.0}, {"x"=0.0, "y"=0.68, "Z"=0.0}, {"x"=0.0, "y"=0.68, "Z"=0.0}, {"x"=0.0, "y"=0.68, "Z"=0.0}, {"x"=0.0, "y"=0.68, "Z"=0.0}, {"x"=0.0, "y"=0.68, "Z"=0.0}, {"x"=0.0, "y"=0.68, "Z"=0.0}, {"x"=0.0, "y"=0.68, "Z"=0.0}, {"x"=0.0, "y"=0.68, "Z"=0.0}, {"x"=0.0, "y"=0.68, "Z"=0.0}, {"x"=0.0, "y"=0.68, "Z"=0.0}, {"x"=0.0, "y"=0.68, "Z"=0.0}, {"x"=0.0, "y"=0.68, "Z"=0.0}, {"x"=0.0, "y"=0.68, "Z"=0.0}, {"x"=0.0, "y"=0.68, "Z"=0.0}, {"x"=0.0, "y"=0.68, "Z"=0.0}, {"x"=0.0, "y"=0.68, "Z"=0.0}, {"x"=0.0, "y"=0.68, "Z"=0.0}, {"x"=0.0, "y"=0.68, "Z"=0.0}, {"x"=0.0, "y"=0.68, "Z"=0.0}, {"x"=0.0, "y"=0.68, "Z"=0.0}, {"x"=0.0, "y"=0.68, "Z"=0.0}, {"x"=0.0, "y"=0.68, "Z"=0.0}, {"x"=0.0, "y"=0.68, "Z"=0.0}, {"x"=0.0, "y"=0.68, "Z"=0.0}, {"x"=0.0, "y"=0.68, "Z"=0.0}, {"x"=0.0, "y"=0.68, "Z"=0.0}, {"x"=0.0, "y"=0.68, "Z"=0.0}, {"x"=0.0, "y"=0.68, "Z"=0.0}, {"x"=0.0, "y"=0.68, "Z"=0.0}, {"x"=0.0, "y"=0.68, "Z"=0.0}, {"x"=0.0, "y"=0.68, "Z"=0.0}, {"x"=0.0, "y"=0.68, "Z"=0.0}, {"x"=0.0, "y"=0.68, "Z"=0.0}, {"x"=0.0, "y"=0.68, "Z"=0.0}, {"x"=0.0, "y"=0.68, "Z"=0.0}, {"x"=0.10283199, "y"=0.61070657, "Z"=-8.989858e-09}, {"x"=0.123903826, "y"=0.5954551, "Z"=-1.0832016e-08}, {"x"=0.12670085, "y"=0.59246206, "Z"=-1.107654e-08}, {"x"=0.120453596, "y"=0.59573895, "Z"=-1.0530388e-08}, {"x"=0.11832927, "y"=0.5961956, "Z"=-1.0344674e-08}, {"x"=0.123528585, "y"=0.59142977, "Z"=-1.0799212e-08}, {"x"=0.11653699, "y"=0.595412, "Z"=-1.0187987e-08}, {"x"=0.112819545, "y"=0.59710395, "Z"=-9.8629975e-09}, {"x"=0.11955698, "y"=0.591078, "Z"=-1.0452003e-08}, {"x"=0.11823877, "y"=0.5909854, "Z"=-1.0336762e-08}, {"x"=0.11930976, "y"=0.58908695, "Z"=-1.0430391e-08}, {"x"=0.12590562, "y"=0.58289814, "Z"=-1.1007018e-08}, {"x"=0.11982058, "y"=0.5864745, "Z"=-1.04750475e-08}, {"x"=0.116135694, "y"=0.5882585, "Z"=-1.0152905e-08}, {"x"=0.11169465, "y"=0.59070665, "Z"=-9.764657e-09}, {"x"=0.11817025, "y"=0.58439773, "Z"=-1.0330771e-08}, {"x"=0.12534976, "y"=0.5773772, "Z"=-1.0958424e-08}, {"x"=0.11859014, "y"=0.5817535, "Z"=-1.0367479e-08}, {"x"=0.0015326833, "y"=0.67871517, "Z"=-1.3399143e-10}, {"x"=0.0015251831, "y"=0.6787062, "Z"=-1.3333575e-10}, {"x"=0.0015176313, "y"=0.6786974, "Z"=-1.3267555e-10}, {"x"=0.0015100281, "y"=0.6786886, "Z"=-1.3201085e-10}, {"x"=0.001502374, "y"=0.6786798, "Z"=-1.313417e-10}, {"x"=0.0014946688, "y"=0.6786711, "Z"=-1.3066809e-10}, {"x"=0.0014869131, "y"=0.6786624, "Z"=-1.2999007e-10}, {"x"=0.0014791071, "y"=0.67865384, "Z"=-1.2930765e-10}, {"x"=0.0014712511, "y"=0.67864525, "Z"=-1.2862086e-10}, {"x"=0.27071887, "y"=0.4277872, "Z"=-2.3666995e-08}, {"x"=0.2721579, "y"=0.42347306, "Z"=-2.37928e-08}, {"x"=0.27066106, "y"=0.42189422, "Z"=-2.3661942e-08}, {"x"=0.26699603, "y"=0.4224071, "Z"=-2.3341533e-08}, {"x"=0.26334623, "y"=0.42295375, "Z"=-2.3022459e-08}, {"x"=0.26469263, "y"=0.4186156, "Z"=-2.3140165e-08}, {"x"=0.26316765, "y"=0.41708028, "Z"=-2.3006846e-08}], 11 "In Range Data":T1(array[cluster])) -> (3 "Obstacle Stop":bool)   [LabVIEW 2019]
uses:
  Ctrl/obstacle_info.ctl
panel:
  out "추가된 배열":bool[](array[boolean])
  out "웨이브폼 차트":cluster{"Point limit":u16, dbl, "x":dbl}(graph)
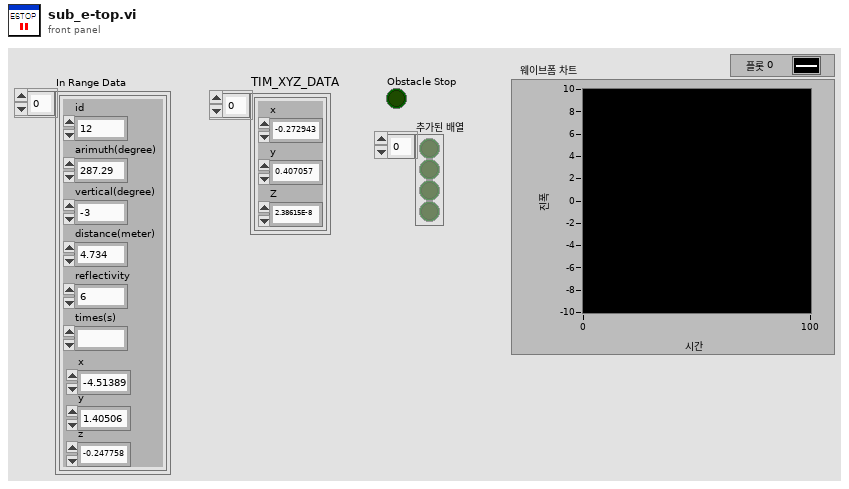
[diagram p1: front panel]
types:
  T1 = cluster{"id":i32, "arimuth(degree)":dbl, "vertical(degree)":dbl, "distance(meter)":dbl, "reflectivity":u8, "times(s)":ext, "x":dbl, "y":dbl, "z":dbl}[]
  T2 = typedef "obstacle_info.ctl" = enum16{"init", "read", "obstacle status in", "write limit", "inrange pt-n"}
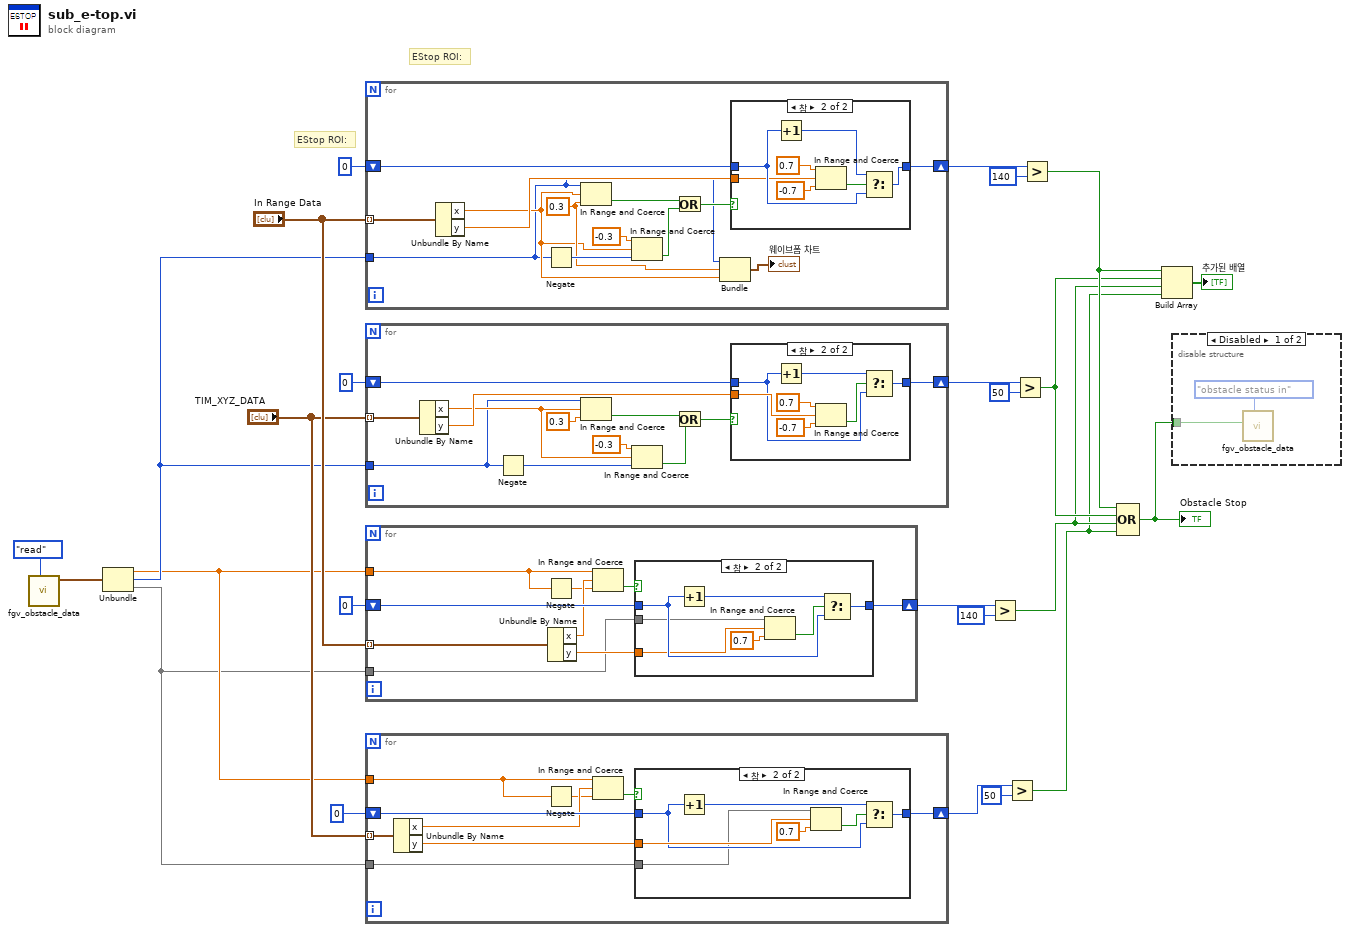
[diagram p0: block diagram]
diagram:
  # "EStop ROI:"
  # "EStop ROI:"
  n1 = call "fgv_obstacle_data.vi"("cmd"=obstacle_info."read") -> ("limit out"=w11:cluster{"RL range":dbl, "Point limit":u16})  [unwired: 7 in, 3 out]
  n2 = Unbundle(w11) -> (w7:dbl, w10:u16, w1)
  n3 = for {
    tunnel: "In Range Data" -> [w38] mode=indexing
    shift-right: [w35] -> w23
    shift-left: 0 -> [w36]
    tunnel: w10 -> [w26]
    w29 = 0.3
    n4 = Unbundle By Name(w38) -> ("x"=w28:dbl, "y"=w37:dbl)
    n5 = Negate(x=w26) -> (-x=w30:i16)
    n6 = In Range and Coerce(upper limit=w26, x=w28, lower limit=w29) -> (In Range?=w33:bool)  [unwired: 1 out]
    n7 = In Range and Coerce(upper limit=-0.3, x=w28, lower limit=w30) -> (In Range?=w32:bool)  [unwired: 1 out]
    n8 = Or(x=w33, y=w32) -> (x .or. y?=w31:bool)
    n9 = Bundle("Point limit"=w26, w29, "x"=w28) -> (→"웨이브폼 차트":cluster{"Point limit":u16, dbl, "x":dbl})  [unwired: 1 in]
    n10 = case shown="참" w31 {
      tunnel: w37 -> [_ w41]
      tunnel: w36 -> [w39 w43]
      tunnel: [w39 w42] -> w35
      frame False {
      }
      frame True {
        n11 = Increment(x=w43) -> (x+1=w44:i32)
        n12 = In Range and Coerce(upper limit=0.7, x=w41, lower limit=-0.7) -> (In Range?=w40:bool)  [unwired: 1 out]
        n13 = Select(t=w44, s=w40, f=w43) -> (s? t:f=w42:i32)
      }
    }
  }
  n14 = for {
    tunnel: "TIM_XYZ_DATA" -> [w58] mode=indexing
    shift-right: [w55] -> w20
    shift-left: 0 -> [w56]
    tunnel: w10 -> [w47]
    n15 = Unbundle By Name(w58) -> ("x"=w52:sgl, "y"=w53:sgl)
    n16 = Negate(x=w47) -> (-x=w48:i16)
    n17 = In Range and Coerce(upper limit=w47, x=w52, lower limit=0.3) -> (In Range?=w51:bool)  [unwired: 1 out]
    n18 = In Range and Coerce(upper limit=-0.3, x=w52, lower limit=w48) -> (In Range?=w50:bool)  [unwired: 1 out]
    n19 = Or(x=w51, y=w50) -> (x .or. y?=w49:bool)
    n20 = case shown="참" w49 {
      tunnel: w53 -> [_ w66]
      tunnel: w56 -> [w59 w61]
      tunnel: [w59 w60] -> w55
      frame False {
      }
      frame True {
        n21 = Increment(x=w61) -> (x+1=w62:i32)
        n22 = In Range and Coerce(upper limit=0.7, x=w66, lower limit=-0.7) -> (In Range?=w63:bool)  [unwired: 1 out]
        n23 = Select(t=w62, s=w63, f=w61) -> (s? t:f=w60:i32)
      }
    }
  }
  n24 = for {
    tunnel: "In Range Data" -> [w75] mode=indexing
    shift-right: [w72] -> w17
    shift-left: 0 -> [w73]
    tunnel: w7 -> [w68]
    tunnel: w1 -> [w67]
    n25 = Negate(x=w68) -> (-x=w69:dbl)
    n26 = Unbundle By Name(w75) -> ("x"=w71:dbl, "y"=w74:dbl)
    n27 = In Range and Coerce(upper limit=w68, x=w71, lower limit=w69) -> (In Range?=w70:bool)  [unwired: 1 out]
    n28 = case shown="참" w70 {
      tunnel: w74 -> [_ w79]
      tunnel: w73 -> [w76 w81]
      tunnel: [w76 w80] -> w72
      tunnel: w67 -> [_ w77]
      frame False {
      }
      frame True {
        n29 = Increment(x=w81) -> (x+1=w82:i32)
        n30 = In Range and Coerce(upper limit=w77, x=w79, lower limit=0.7) -> (In Range?=w78:bool)  [unwired: 1 out]
        n31 = Select(t=w82, s=w78, f=w81) -> (s? t:f=w80:i32)
      }
    }
  }
  n32 = for {
    tunnel: "TIM_XYZ_DATA" -> [w92] mode=indexing
    shift-right: [w90] -> w14
    shift-left: 0 -> [w91]
    tunnel: w7 -> [w85]
    tunnel: w1 -> [w84]
    n33 = Unbundle By Name(w92) -> ("x"=w88:sgl, "y"=w89:sgl)
    n34 = Negate(x=w85) -> (-x=w86:dbl)
    n35 = In Range and Coerce(upper limit=w85, x=w88, lower limit=w86) -> (In Range?=w87:bool)  [unwired: 1 out]
    n36 = case shown="참" w87 {
      tunnel: w89 -> [_ w100]
      tunnel: w91 -> [w93 w96]
      tunnel: [w93 w95] -> w90
      tunnel: w84 -> [_ w94]
      frame False {
      }
      frame True {
        n37 = Increment(x=w96) -> (x+1=w97:i32)
        n38 = In Range and Coerce(upper limit=w94, x=w100, lower limit=0.7) -> (In Range?=w98:bool)  [unwired: 1 out]
        n39 = Select(t=w97, s=w98, f=w96) -> (s? t:f=w95:i32)
      }
    }
  }
  n40 = Greater?(x=w17, y=140) -> (0:w4:bool)
  n41 = Greater?(x=w14, y=50) -> (0:w3:bool)
  n42 = Greater?(x=w20, y=50) -> (0:w5:bool)
  n43 = Greater?(x=w23, y=140) -> (0:w6:bool)
  n44 = Compound Arithmetic op=OR(w6, w5, w4, w3) -> (w8:bool)
  "Obstacle Stop" <- w8
  n45 = Build Array(w6, w5, w4, w3) -> (→"추가된 배열":bool[])
  n46 = disable-structure shown="Disabled" {
    disable-tunnel: w8 -> [w101 _]
    frame Disabled {
      n47 = call "fgv_obstacle_data.vi"("cmd"=obstacle_info."obstacle status in", "obstacle in"=w101) -> ()  [unwired: 6 in, 4 out]
    }
    frame Enabled {
    }
  }
